vi "Test_Werte.vi"(0 "time":sgl, 1 "frei_2":sgl, 2 "frei_1":sgl, 4 "MotorSpeed":sgl, 5 "Beschleunigung":sgl, 6 "MototPos":sgl, 7 "Gyro Speed":sgl, 8 "MotorSumme":sgl, 9 "Reglerausgang":sgl, 10 "FilterWinkel":sgl, 11 "Gyro Winkel":sgl) -> (3 "concatenated string":string)   [LabVIEW 2009]
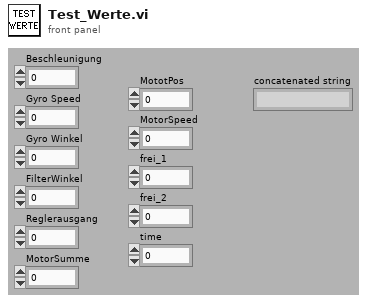
[diagram p1: front panel]
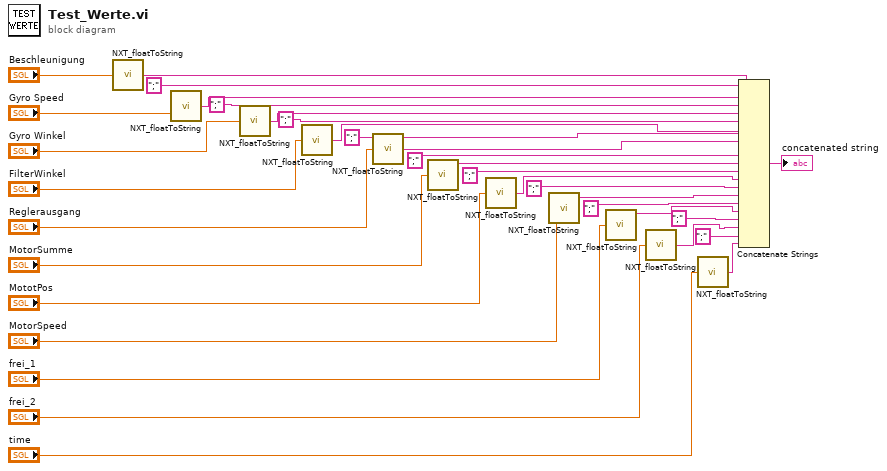
[diagram p0: block diagram]
diagram:
  n1 = call <vilib>:"NXT_floatToString.vi"("number"="Beschleunigung") -> ("string"=w33:string)
  n2 = call <vilib>:"NXT_floatToString.vi"("number"="Gyro Speed") -> ("string"=w31:string)
  n3 = call <vilib>:"NXT_floatToString.vi"("number"="Gyro Winkel") -> ("string"=w29:string)
  n4 = call <vilib>:"NXT_floatToString.vi"("number"="FilterWinkel") -> ("string"=w27:string)
  n5 = call <vilib>:"NXT_floatToString.vi"("number"="Reglerausgang") -> ("string"=w25:string)
  n6 = call <vilib>:"NXT_floatToString.vi"("number"="MotorSumme") -> ("string"=w22:string)
  n7 = call <vilib>:"NXT_floatToString.vi"("number"="MototPos") -> ("string"=w21:string)
  n8 = call <vilib>:"NXT_floatToString.vi"("number"="MotorSpeed") -> ("string"=w18:string)
  n9 = call <vilib>:"NXT_floatToString.vi"("number"="frei_1") -> ("string"=w17:string)
  n10 = call <vilib>:"NXT_floatToString.vi"("number"="frei_2") -> ("string"=w13:string)
  n11 = call <vilib>:"NXT_floatToString.vi"("number"="time") -> ("string"=w14:string)
  n12 = Concatenate Strings(w33, ";" ("string"), w31, ";" ("string"), w29, ";" ("string"), w27, ";" ("string"), w25, ";" ("string"), w22, ";" ("string"), w21, ";" ("string"), w18, ";" ("string"), w17, ";" ("string"), w13, ";" ("string"), w14) -> (→"concatenated string":string)
